vi "lsl set child value.vi"(8 "error in (no error)":errorcluster, 9 "value":string, 10 "name":string, 11 "e":cluster{}) -> (0 "error out":errorcluster, 2 "function return":i32, 3 "e out":cluster{})   [LabVIEW 2018, in "liblsl-LabVIEW.lvlib"]
doc: "extern LIBLSL_C_API int32_t lsl_set_child_value(lsl_xml_ptr e, const char *name, const char *value);"
uses:
  <userlib>/liblsl-LabVIEW/liblsl-LabVIEW.lvlib
  <userlib>/liblsl-LabVIEW/liblsl64.dll
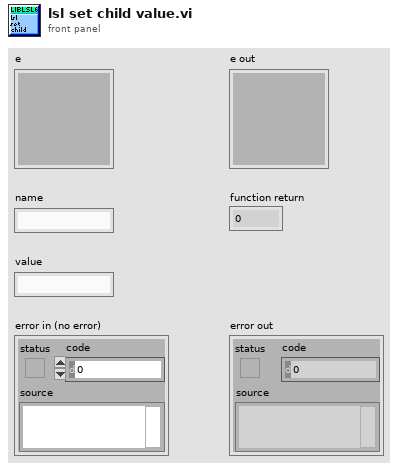
[diagram p1: front panel]
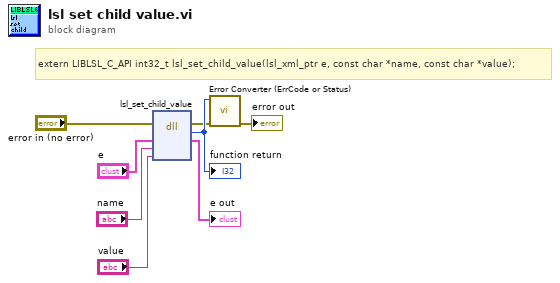
[diagram p0: block diagram]
diagram:
  # "extern LIBLSL_C_API int32_t lsl_set_child_value(lsl_xml_ptr e, const char *name, const char *value);"
  n1 = dll-call lib="C:/Program Files/National Instruments/LabVIEW 2018/user.lib/liblsl-LabVIEW/liblsl64.*" fn="lsl_set_child_value"(error in="error in (no error)", "e"="e", "name"="name", "value"="value") -> (error out=w2:errorcluster, w8:i32, "e"=→"e out":cluster{})  [unwired: 4 in, 1 out]
  "function return" <- w8
  n2 = call <userlib>:"Error Converter (ErrCode or Status).vi"("error in (no error)"=w2, "error code"=w8) -> ("error out"=→"error out":errorcluster)  [unwired: 9 in]
